vi "Obtain AnalogIn.vi"(7 "ADC #":T1=-1, 8 "error in (no error)":errorcluster, 11 "Session in":refnum<class "Session.lvclass">) -> (0 "error out":errorcluster, 2 "AnalogIn":refnum<class "AI.lvclass">, 3 "Session out":refnum<class "Session.lvclass">)   [LabVIEW 2020, in "CTI.lvlib" / "Session.lvclass"]
uses:
  Session.lvclass
  Session.lvclass/Session.ctl
  AI/AI.lvclass
  GPIO/GPIO.lvclass
  ADC Number.ctl
  CTI.lvlib
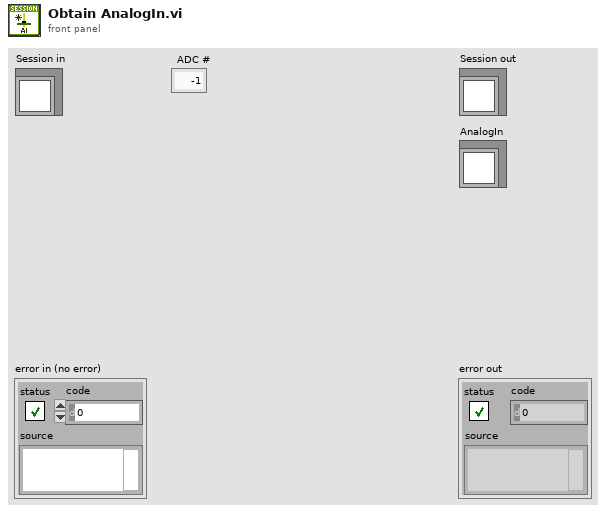
[diagram p1: front panel]
types:
  T1 = typedef "CTI.lvlib/ADC Number.ctl" = i8
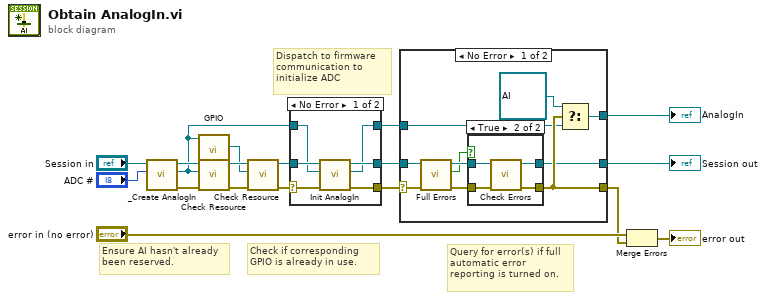
[diagram p0: block diagram]
diagram:
  # "Query for error(s) if full automatic error reporting is turned on."
  # "Dispatch to firmware communication to initialize ADC"
  # "Ensure AI hasn't already been reserved."
  # "Check if corresponding GPIO is already in use."
  n1 = call "_Create AnalogIn.vi"("ADC #"="ADC #", "Session in"="Session in") -> ("error out"=w6:errorcluster, "AnalogIn out"=w2:refnum<class "AI.lvclass">, "Session out"=w5:refnum<class "Session.lvclass">)  [unwired: 7 in]
  n2 = call "GPIO.vi"("AnalogIn in"=w2) -> ("GPIO"=w1:refnum<class "GPIO.lvclass">)  [unwired: 10 in]
  n3 = call "Check Resource.vi"("error in (no error)"=w6, "Resource"=w2, "Session in"=w5) -> ("error out"=w4:errorcluster, "Session out"=w3:refnum<class "Session.lvclass">)  [unwired: 7 in]
  n4 = call "Check Resource.vi"("error in (no error)"=w4, "Resource"=w1, "Session in"=w3) -> ("error out"=w10:errorcluster, "Session out"=w9:refnum<class "Session.lvclass">)  [unwired: 7 in]
  n5 = case shown="No Error" w10 {
    selector: w10 -> [w23 w25]
    tunnel: w9 -> [w24 w26]
    tunnel: w2 -> [w22 _]
    tunnel: [w19 _] -> w16
    tunnel: [w21 w25] -> w18
    tunnel: [w20 w26] -> w17
    frame No Error {
      n6 = call-dynamic "Init AnalogIn.vi"("error in (no error)"=w23, "AnalogIn In"=w22, "Session in"=w24) -> ("error out"=w21:errorcluster, "AnalogIn"=w19:refnum<class "AI.lvclass">, "Session out"=w20:refnum<class "Session.lvclass">)  [unwired: 6 in]
    }
    frame Error {
    }
  }
  n7 = case shown="No Error" w18 {
    selector: w18 -> [w34 w44]
    tunnel: w17 -> [w35 w43]
    tunnel: w16 -> [w29 _]
    tunnel: [w28 _] -> w15
    tunnel: [w36 w44] -> w12
    tunnel: [w30 w43] -> w14
    frame No Error {
      n8 = call "Full Errors.vi"("error in (no error)"=w34, "Session in"=w35) -> ("error out"=w32:errorcluster, "Full Errors"=w31:bool, "Session out"=w33:refnum<class "Session.lvclass">)  [unwired: 7 in]
      n9 = case shown="True" w31 {
        tunnel: w33 -> [w38 w42]
        tunnel: w32 -> [w37 w41]
        tunnel: [w37 w40] -> w36
        tunnel: [w38 w39] -> w30
        frame False {
        }
        frame True {
          n10 = call "Check Errors.vi"("error in (no error)"=w41, "Session in"=w42) -> ("error out"=w40:errorcluster, "Session out"=w39:refnum<class "Session.lvclass">)  [unwired: 8 in]
        }
      }
      n11 = Select(t=refnum<class "AI.lvclass"> refnum, s=w36, f=w29) -> (s? t:f=w28:refnum<class "AI.lvclass">)
    }
    frame Error {
    }
  }
  "Session out" <- w14
  "AnalogIn" <- w15
  n12 = Merge Errors("error in (no error)", w12) -> (→"error out":errorcluster)
